vi "ScanDelay_FTIR_AcquireInterferogram_DAQmx.vi"(9 "Sampling rate":dbl=250000.0, 10 "Time per acquisiton (s)":dbl=0.125) -> (3 "Output V-d array":dbl[][](array[numeric]))   [LabVIEW 2022 SP3]
uses:
  <vilib>/DAQmx/read.llb/DAQmx Read (Analog 2D DBL NChan NSamp).vi
panel:
  in  "Trigger Terminal":tag
  in  "Channels to read":tag
  in  "Plot?":bool
  out "Acquisition cycle":dbl[][](graph)
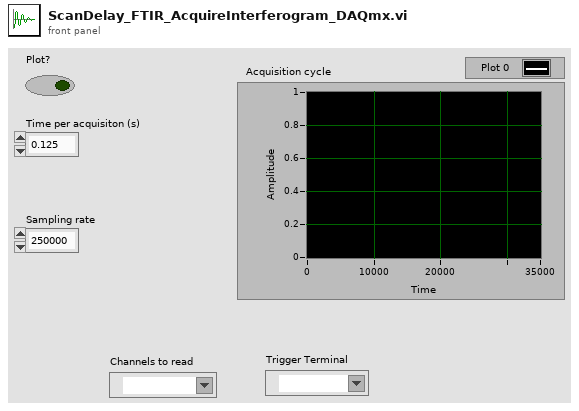
[diagram p1: front panel]
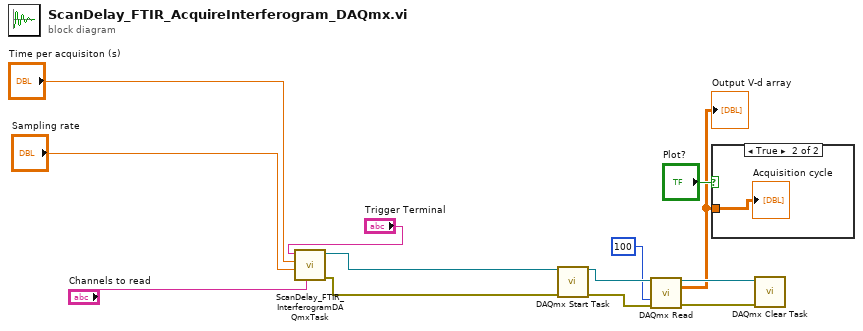
[diagram p0: block diagram]
diagram:
  n1 = call "ScanDelay_FTIR_InterferogramDAQmxTask.vi"("First clear existing DAQmx tasks"="Channels to read", "Sampling rate"="Sampling rate", "Time per acquisiton (s)"="Time per acquisiton (s)", "Trigger Terminal"="Trigger Terminal") -> ("error out"=w8:errorcluster, "Refnum out"=w1:refnum<k21>)  [unwired: 6 in]
  n2 = call <vilib>:"DAQmx Start Task.vi"("task/channels in"=w1, "error in"=w8) -> ("task out"=w7:refnum<k21>, "error out"=w6:errorcluster)  [unwired: 12 in]
  n3 = call-poly <vilib>:"DAQmx Read.vi"("task/channels in"=w7, "timeout"=100, "error in"=w6) -> ("task out"=w4:refnum<k21>, "data"=w2:dbl[][], "error out"=w3:errorcluster)  [unwired: 10 in]
  "Output V-d array" <- w2
  n4 = case shown="True" "Plot?" {
    tunnel: w2 -> [_ w14]
    frame False {
    }
    frame True {
      "Acquisition cycle" <- w14
    }
  }
  n5 = call <vilib>:"DAQmx Clear Task.vi"("task in"=w4, "error in"=w3) -> ()  [unwired: 13 in, 1 out]
